vi "FFT and INV FFT filter.vi"(3 "Desired cut off Freq":dbl step=10.0, 4 "Average Sampling Rate":dbl, 5 "Signal":dbl[](array[numeric]) format="%0.2f") -> (2 "Filtered Sgnal":dbl[](array[numeric]))   [LabVIEW 2022 SP3]
uses:
  <vilib>/Analysis/baseanly.llb/Mean (DBL).vi
  <vilib>/Analysis/2dsp.llb/Real FFT.vi
  <vilib>/Analysis/2dsp.llb/Inverse Real FFT.vi
  <vilib>/Analysis/NI_AALBase.lvlib
  <vilib>/Analysis/NI_AALPro.lvlib
panel:
  out "Delta F":dbl
  out "Waveform Graph":dbl[][](graph)
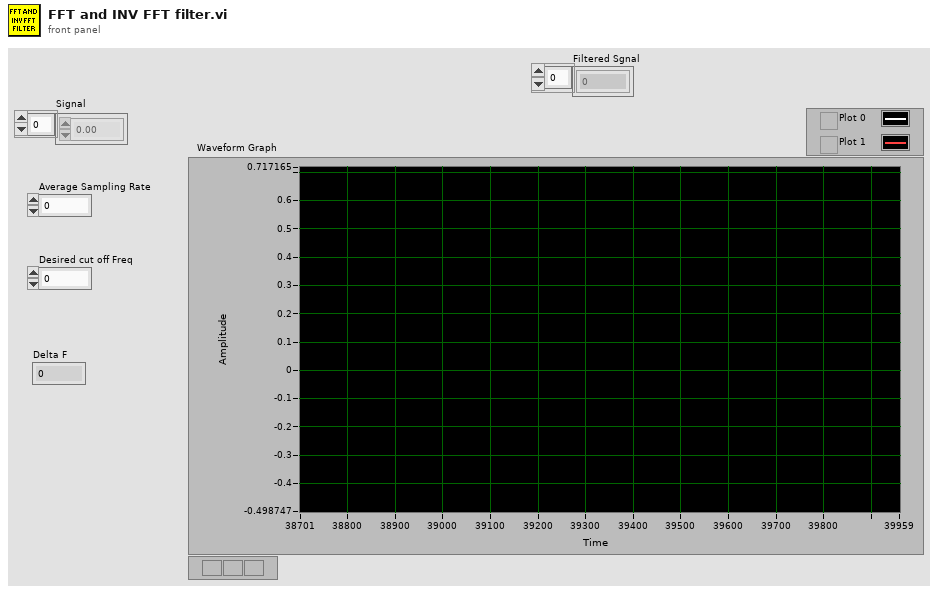
[diagram p1: front panel]
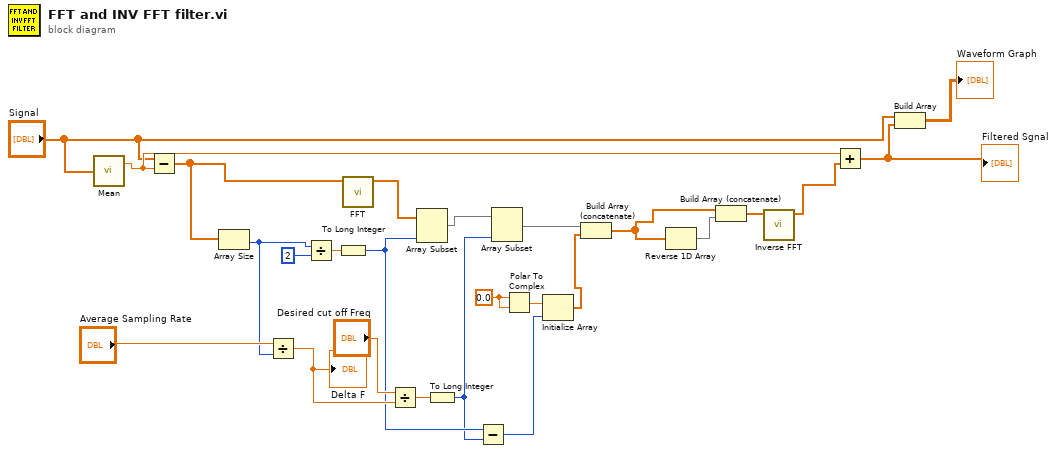
[diagram p0: block diagram]
diagram:
  w18 = 0.0 ("r")
  n1 = call-poly <vilib>:"Mean.vi"("X"="Signal") -> ("mean"=w7:dbl)  [unwired: 1 out]
  n2 = Subtract(x="Signal", y=w7) -> (x-y=w23:dbl[])
  n3 = Array Size(array=w23) -> (size(s)=w21:i32)
  n4 = Divide(x="Average Sampling Rate", y=w21) -> (x/y=w19:dbl)
  "Delta F" <- w19
  n5 = Divide(x=w21, y=2) -> (x/y=w16:dbl)
  n6 = To Long Integer(number=w16) -> (32bit integer=w15:i32)
  n7 = call-poly <vilib>:"FFT.vi"("X"=w23) -> ("FFT {X}"=w25:cdb[])  [unwired: 9 in, 1 out]
  n8 = Divide(x="Desired cut off Freq", y=w19) -> (x/y=w17:dbl)
  n9 = Array Subset(array=w25, length=w15) -> (w3:cdb[])  [unwired: 1 in]
  n10 = To Long Integer(number=w17) -> (32bit integer=w14:i32)
  n11 = Subtract(x=w15, y=w14) -> (x-y=w13:i32)
  n12 = Array Subset(array=w3, length=w14) -> (w11:cdb[])  [unwired: 1 in]
  n13 = Polar To Complex(1:w18, 2:w18) -> (0:w12:cdb)
  n14 = Initialize Array(w12, w13) -> (w10:cdb[])
  n15 = Build Array (concatenate)(w11, w10) -> (w1:cdb[])
  n16 = Reverse 1D Array(array=w1) -> (reversed array=w9:cdb[])
  n17 = Build Array (concatenate)(w1, w9) -> (w2:cdb[])
  n18 = call-poly <vilib>:"Inverse FFT.vi"("FFT {X}"=w2) -> ("X"=w8:dbl[])  [unwired: 9 in, 1 out]
  n19 = Add(x=w7, y=w8) -> (x+y=w5:dbl[])
  "Filtered Sgnal" <- w5
  n20 = Build Array("Signal", w5) -> (→"Waveform Graph":dbl[][])
